vi "ExtraDownsample_2channel.vi"(6 "reset":bool, 7 "Set downsample":bool, 8 "valid in":bool, 9 "Downsample":fxp<+,8,8>, 10 "CIC Gain":fxp<+/-,32,1>=0.00390625 format="%#_32g", 11 "Data in":fxp<+/-,16,14>[](array[numeric])=[0.0, 0.0, 0.0, 0.0]) -> (0 "valid out":bool, 3 "Element":u64)   [LabVIEW 2013]
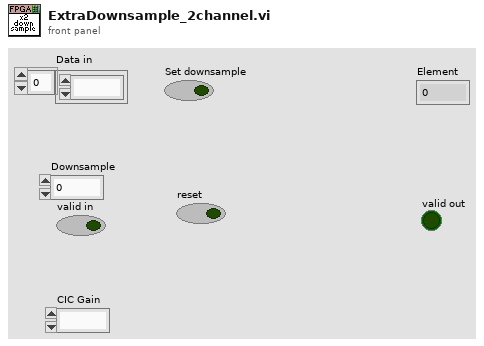
[diagram p1: front panel]
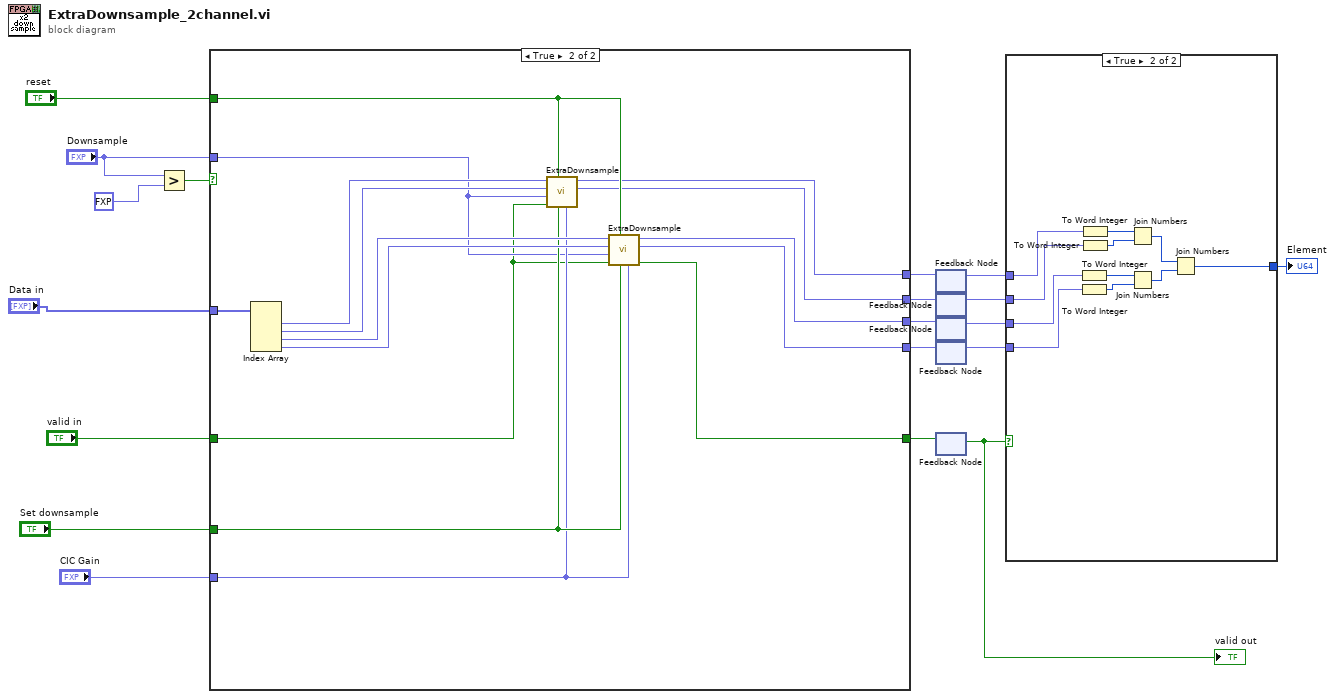
[diagram p0: block diagram]
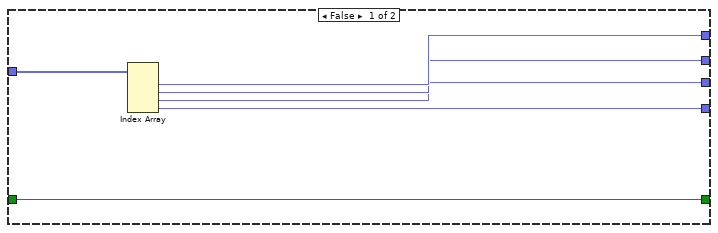
[diagram p3: hidden frame]
diagram:
  n1 = Greater?(x="Downsample", y=fxp<+,8,8> 1.0) -> (0:w18:bool)
  n2 = case shown="True" w18 {
    tunnel: "Data in" -> [w24 w40]
    tunnel: "Downsample" -> [_ w32]
    tunnel: "valid in" -> [w25 w31]
    tunnel: "reset" -> [_ w35]
    tunnel: "Set downsample" -> [_ w34]
    tunnel: "CIC Gain" -> [_ w33]
    tunnel: [w25 w30] -> w10
    tunnel: [w23 w26] -> w6
    tunnel: [w22 w27] -> w4
    tunnel: [w21 w28] -> w2
    tunnel: [w20 w29] -> w8
    frame False {
      n3 = Index Array(array=w24) -> (element #1=w23:fxp<+/-,16,14>, element #2=w22:fxp<+/-,16,14>, element #3=w21:fxp<+/-,16,14>, element #4=w20:fxp<+/-,16,14>)  [unwired: 4 in]
    }
    frame True {
      n4 = Index Array(array=w40) -> (element #1=w39:fxp<+/-,16,14>, element #2=w38:fxp<+/-,16,14>, element #3=w37:fxp<+/-,16,14>, element #4=w36:fxp<+/-,16,14>)  [unwired: 4 in]
      n5 = call "ExtraDownsample.vi"("CIC Gain"=w33, "Set downsample"=w34, "reset"=w35, "valid in"=w31, "Downsample"=w32, "I in"=w38, "Q in"=w39) -> ("Q out"=w27:fxp<+/-,16,14>, "I out"=w26:fxp<+/-,16,14>)  [unwired: 2 in, 1 out]
      n6 = call "ExtraDownsample.vi"("CIC Gain"=w33, "Set downsample"=w34, "reset"=w35, "valid in"=w31, "Downsample"=w32, "I in"=w36, "Q in"=w37) -> ("valid out"=w30:bool, "Q out"=w29:fxp<+/-,16,14>, "I out"=w28:fxp<+/-,16,14>)  [unwired: 2 in]
    }
  }
  n7 = feedback #1() -> (w5:fxp<+/-,16,14>)  [unwired: 1 in]
  n8 = feedback-in #1(w6) -> ()
  n9 = feedback #2() -> (w3:fxp<+/-,16,14>)  [unwired: 1 in]
  n10 = feedback-in #2(w4) -> ()
  n11 = feedback #3() -> (w1:fxp<+/-,16,14>)  [unwired: 1 in]
  n12 = feedback-in #3(w2) -> ()
  n13 = feedback #4() -> (w7:fxp<+/-,16,14>)  [unwired: 1 in]
  n14 = feedback-in #4(w8) -> ()
  n15 = feedback #5() -> (w9:bool)  [unwired: 1 in]
  "valid out" <- w9
  n16 = feedback-in #5(w10) -> ()
  n17 = case shown="True" w9 {
    tunnel: [_ w45] -> w11
    tunnel: w7 -> [_ w44]
    tunnel: w5 -> [_ w43]
    tunnel: w3 -> [_ w42]
    tunnel: w1 -> [_ w41]
    frame False {
    }
    frame True {
      n18 = To Word Integer(number=w41) -> (16bit integer=w49:i16)
      n19 = To Word Integer(number=w44) -> (16bit integer=w48:i16)
      n20 = To Word Integer(number=w43) -> (16bit integer=w50:i16)
      n21 = To Word Integer(number=w42) -> (16bit integer=w51:i16)
      n22 = Join Numbers(hi=w50, lo=w51) -> ((hi.lo)=w47:u32)
      n23 = Join Numbers(hi=w49, lo=w48) -> ((hi.lo)=w46:u32)
      n24 = Join Numbers(hi=w47, lo=w46) -> ((hi.lo)=w45:u64)
    }
  }
  "Element" <- w11
